vi "simple manipulate.vi"() -> ()   [LabVIEW 2013, in "libusvlv.lvlib"]
uses:
  libusvlv.lvlib
  UsbCom.dll
panel:
  in  "?":bool
  in  "read ep":i32=129 format="%x"
  out "DISPLAY":string
  in  "COMMAND":string
  in  "wirte ep":i32=3 format="%x"
  out "flag":u32
  in  "index":i32
  in  "vid":u32=21317 format="%x"
  in  "pid":u32=4660 format="%x"
  in  "?":bool
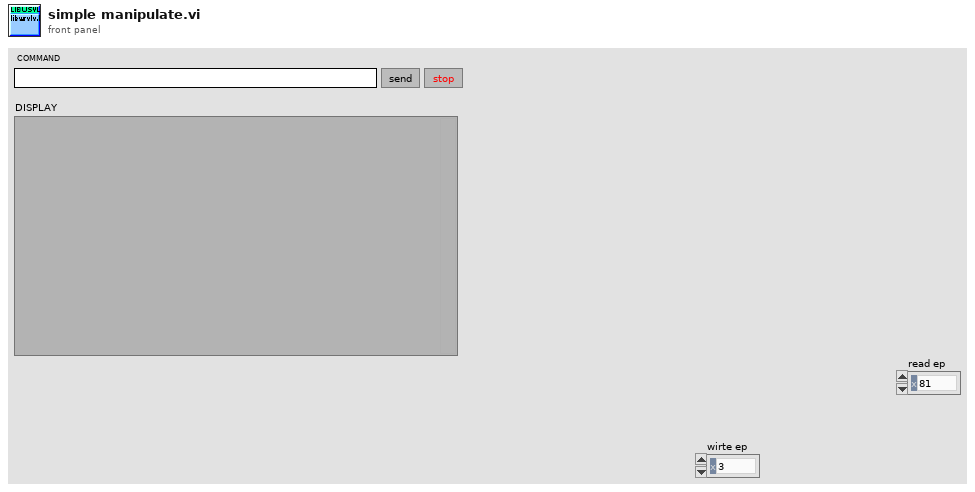
[diagram p1: front panel]
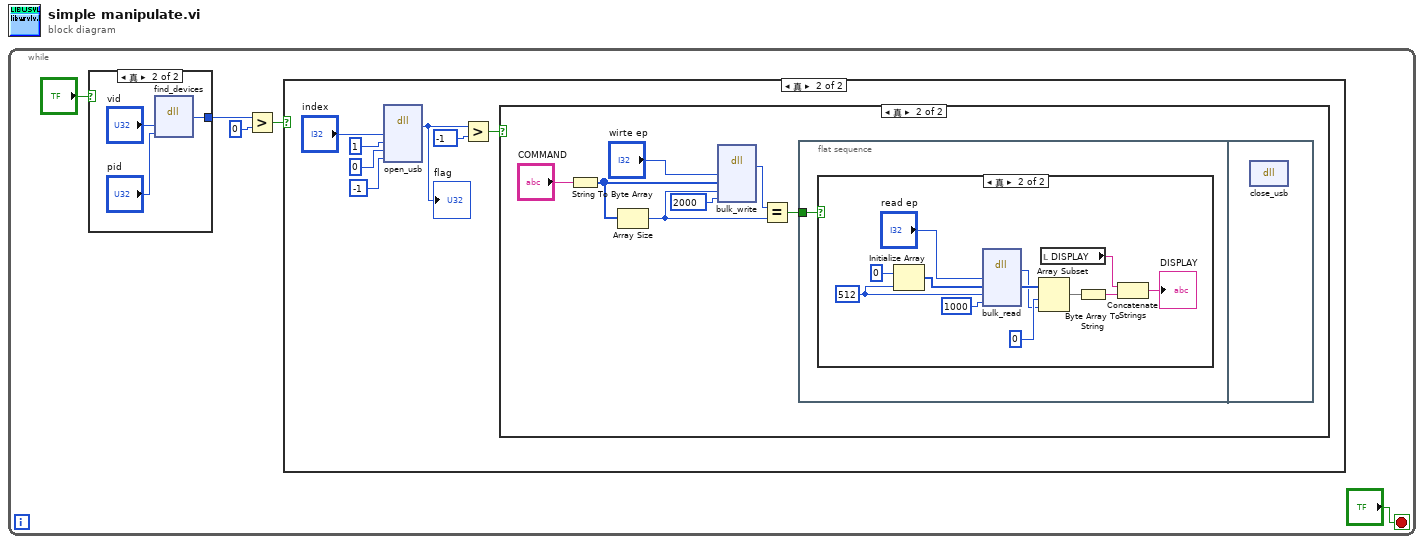
[diagram p0: block diagram]
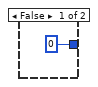
[diagram p5: hidden frame]
diagram:
  n1 = while {
    stop <- "?" stop-if-true
    n2 = case shown="真" "?" {
      tunnel: [0 w34] -> w3
      frame False {
      }
      frame True {
        n3 = dll-call lib="E:/libusvlv/UsbCom.dll" fn="find_devices"("vid"="vid", "pid"="pid") -> ("num"=w34:i32)  [unwired: 5 in, 2 out]
      }
    }
    n4 = Greater?(x=w3, y=0) -> (0:w2:bool)
    n5 = case shown="真" w2 {
      frame False {
      }
      frame True {
        n6 = dll-call lib="E:/libusvlv/UsbCom.dll" fn="open_usb"("idx"="index", "conf"=1, "iface"=0, "altiface"=-1) -> ("返回类型"=w12:i32)  [unwired: 7 in, 2 out]
        "flag" <- w12
        n7 = Greater?(x=w12, y=-1) -> (0:w6:bool)
        n8 = case shown="真" w6 {
          frame False {
          }
          frame True {
            n9 = String To Byte Array(string="COMMAND") -> (unsigned byte array=w17:u8[])
            n10 = Array Size(array=w17) -> (size(s)=w18:i32)
            n11 = dll-call lib="E:/libusvlv/UsbCom.dll" fn="bulk_write"("ep"="wirte ep", "bytes"=w17, "size"=w18, "timeout"=2000) -> ("size"=w19:i32)  [unwired: 6 in, 3 out]
            n12 = Equal?(x=w19, y=w18) -> (x = y?=w13:bool)
            n13 = flat-sequence {
              tunnel: w13 -> [w20]
              frame #0 {
                n14 = case shown="真" w20 {
                  frame False {
                  }
                  frame True {
                    w22 = 512
                    n15 = Initialize Array(0, w22) -> (w31:i32[])
                    n16 = dll-call lib="E:/libusvlv/UsbCom.dll" fn="bulk_read"("ep"="read ep", "bytes"=w31, "size"=w22, "timeout"=1000) -> ("返回类型"=w21:i32, "bytes"=w25:i8[])  [unwired: 6 in, 2 out]
                    n17 = Array Subset(array=w25, index=0, length=w21) -> (w24:i8[])
                    n18 = local read "DISPLAY"() -> (w28:string)
                    n19 = Byte Array To String(unsigned byte array=w24) -> (string=w27:string)
                    n20 = Concatenate Strings(w28, w27) -> (→"DISPLAY":string)
                  }
                }
              }
              frame #1 {
                n21 = dll-call lib="E:/libusvlv/UsbCom.dll" fn="close_usb"() -> ()  [unwired: 3 in, 3 out]
              }
            }
          }
        }
      }
    }
  }
